vi "Logging Message Loop.vi"(8 "error in (no error)":errorcluster, 10 "Data Queue":refnum<queue>, 11 "Message Queues":T1) -> (0 "error out":errorcluster)   [LabVIEW 2016, in "Logging.lvlib"]
doc: "The message loop subVI to handle messages pertaining to logging data."
uses:
  Logging.lvlib
  support/Message Queue/All Message Queues.ctl
  support/Message Queue/Message Cluster.ctl
  Logging Configuration.ctl
  Logging State.ctl
  support/Message Queue/Enqueue Message (Single).vi
  <vilib>/Utility/error.llb/Error Cluster From Error Code.vi
  <vilib>/ErrorRing/Error Ring.xnode
  support/Message Queue/Message Queue.lvlib
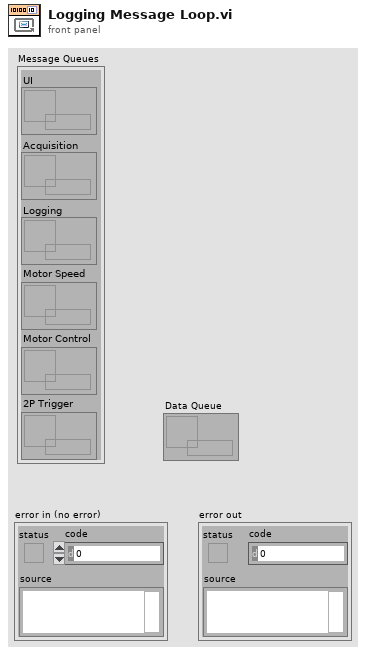
[diagram p1: front panel]
types:
  T1 = typedef "Message Queue.lvlib/All Message Queues.ctl" = cluster{"UI":refnum<queue>, "Acquisition":refnum<queue>, "Logging":refnum<queue>, "Motor Speed":refnum<queue>, "Motor Control":refnum<queue>, "2P Trigger":refnum<queue>}
  T2 = typedef "Logging.lvlib/Logging State.ctl" = cluster{"State":enum16{"Logging", "Not Logging", "Idle"}, "Samples to Save":u32, "Force Trigger":bool}
  T3 = typedef "Logging.lvlib/Logging Configuration.ctl" = cluster{"Log File Base Path":path, "TDMS File Reference":refnum<k34>, "Samples to Save":u32, "Trigger - Time":u32, "Trigger - Threshold":dbl, "Trigger - Channel":u32, "Enable Time Trigger":bool, "Enable Threshold Trigger":bool, "Always Log":bool}
  T4 = enum16{"open", "open or create", "create or replace", "create", "open (read-only)"}
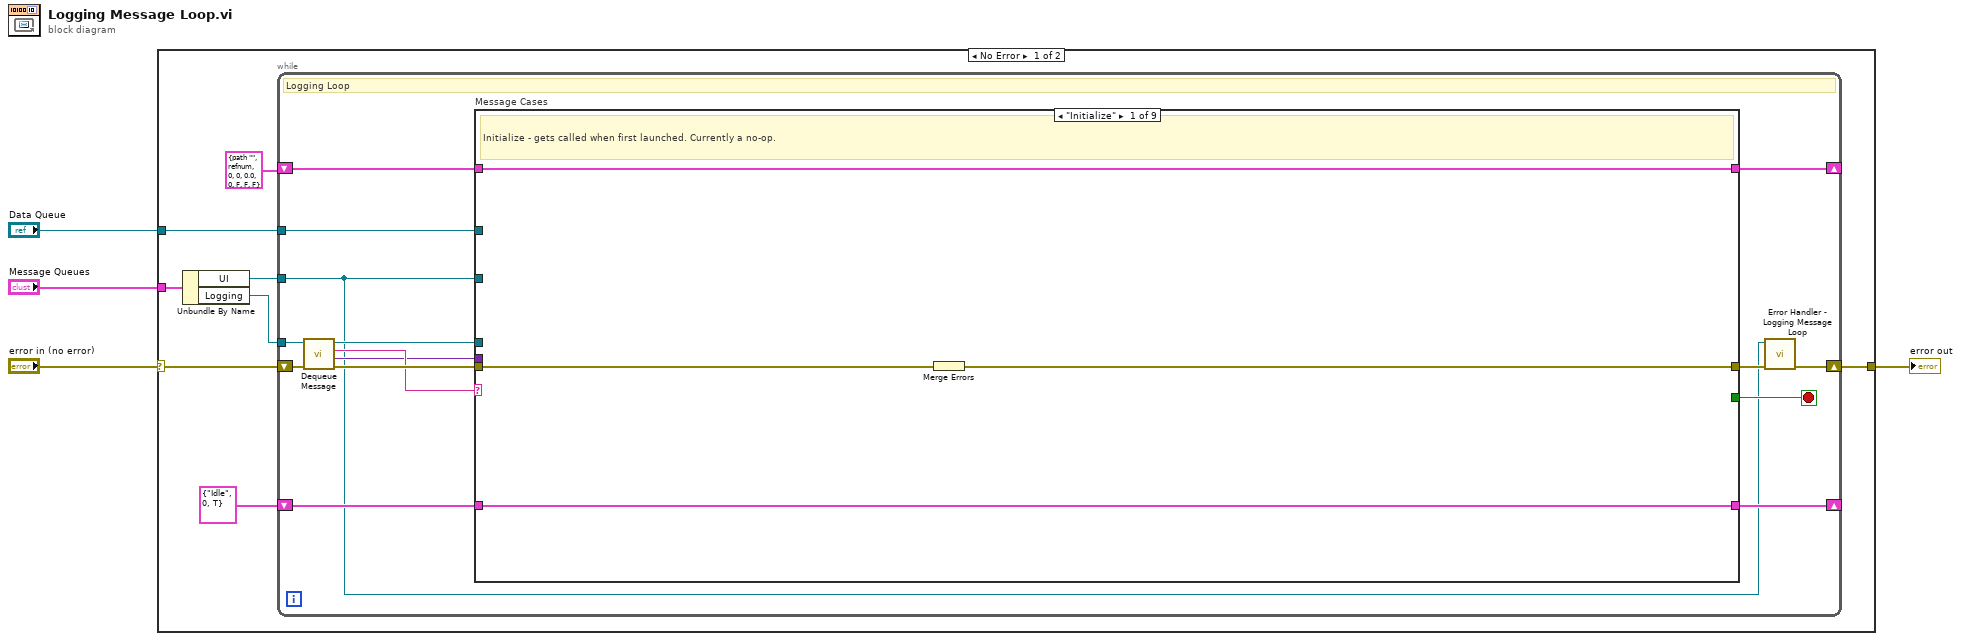
[diagram p0: block diagram]
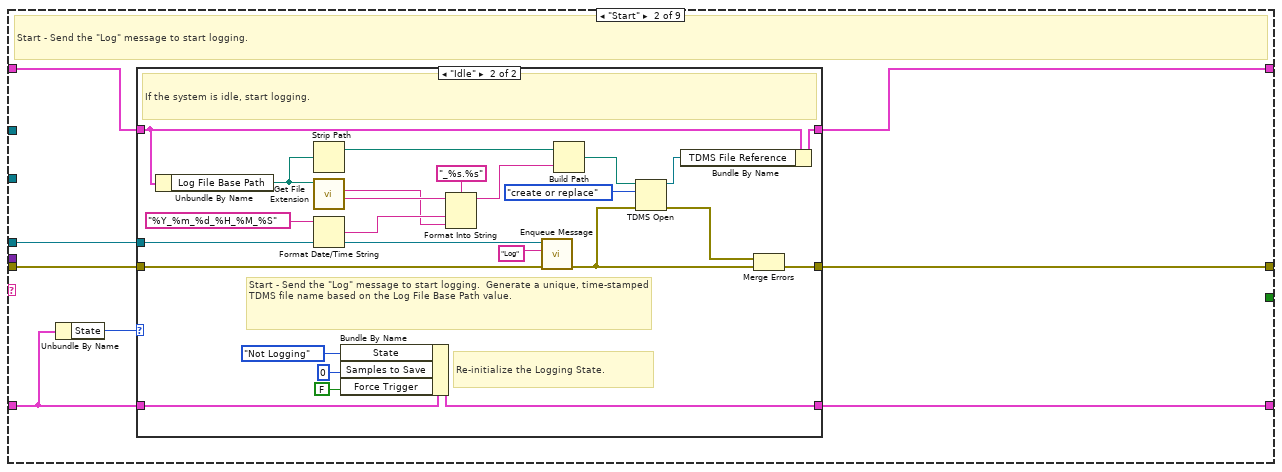
[diagram p2: hidden frame]
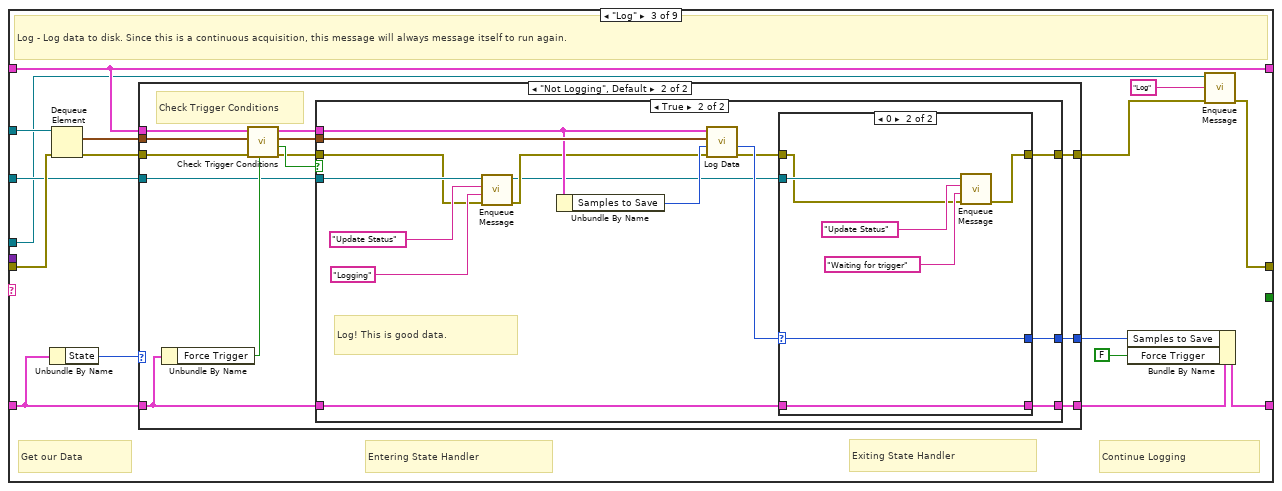
[diagram p4: hidden frame]
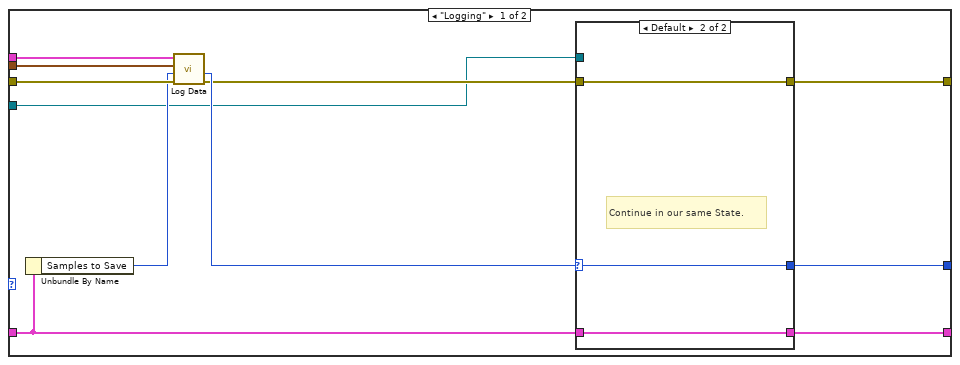
[diagram p5: hidden frame]
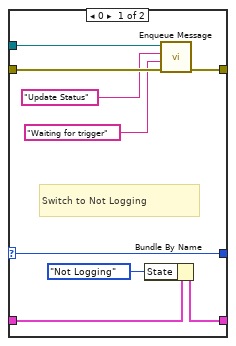
[diagram p6: hidden frame]
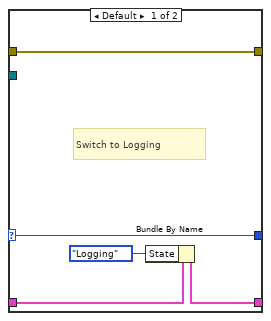
[diagram p8: hidden frame]
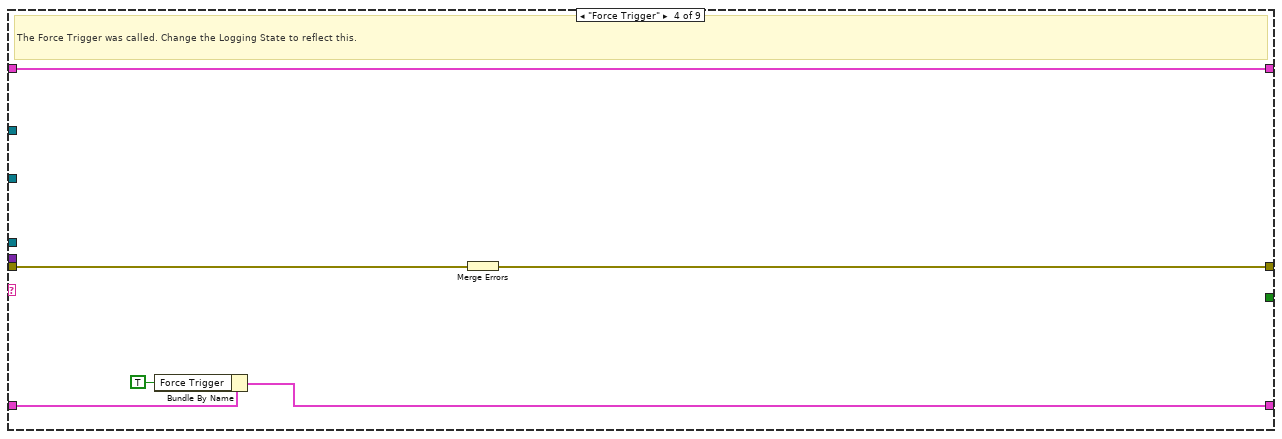
[diagram p9: hidden frame]
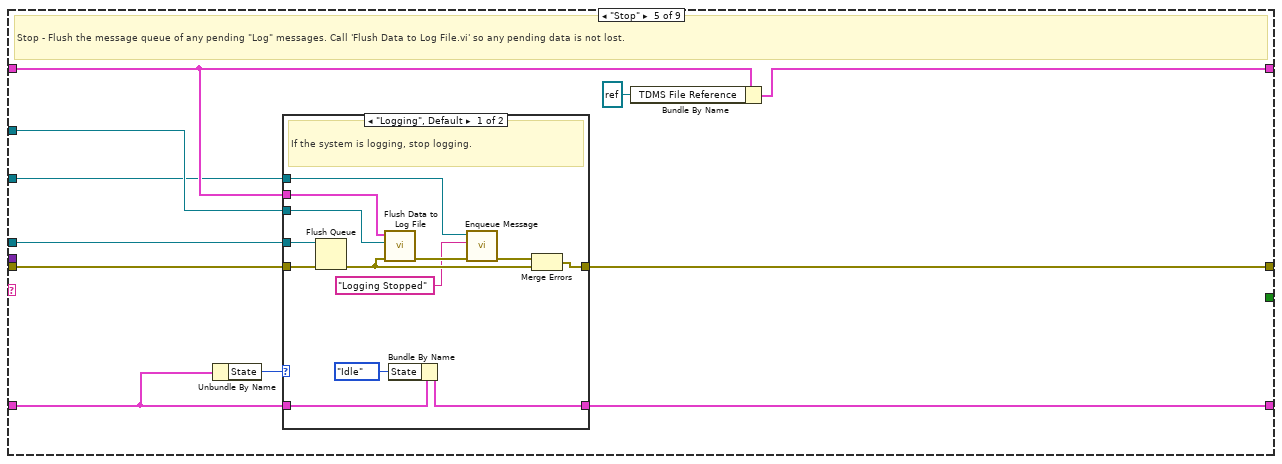
[diagram p10: hidden frame]
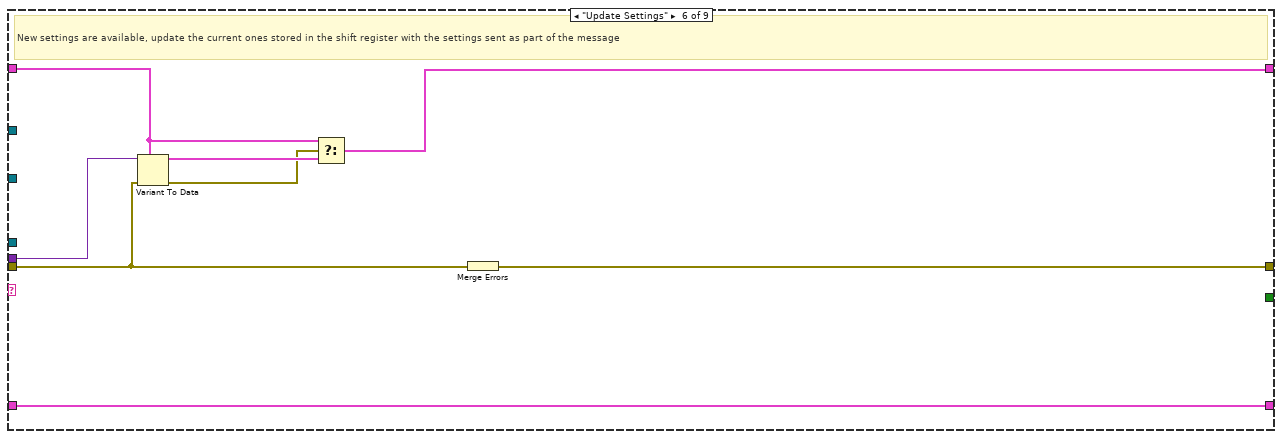
[diagram p12: hidden frame]
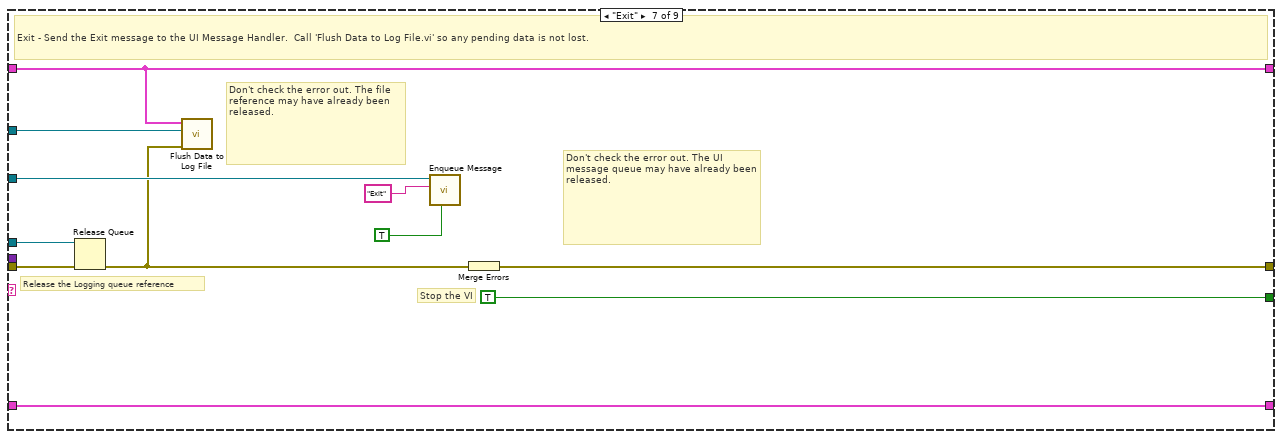
[diagram p13: hidden frame]
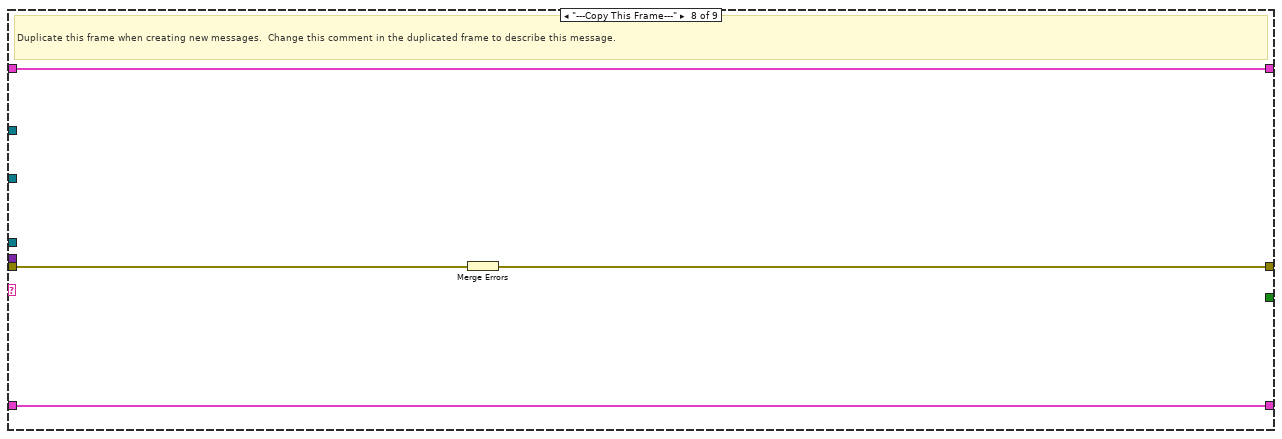
[diagram p14: hidden frame]
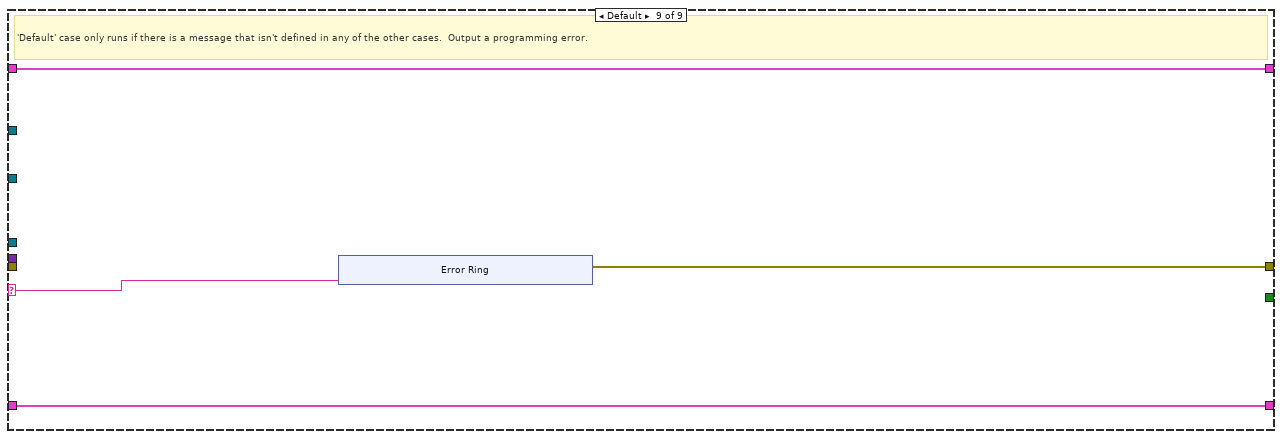
[diagram p15: hidden frame]
diagram:
  n1 = case shown="No Error" "error in (no error)" {
    selector: "error in (no error)" -> [w8 w214]
    tunnel: "Message Queues" -> [w12 _]
    tunnel: [w10 w214] -> w3
    tunnel: "Data Queue" -> [w7 _]
    frame No Error {
      n2 = Unbundle By Name(w12) -> ("UI"=w6:refnum<queue>, "Logging"=w11:refnum<queue>)
      n3 = while {
        tunnel: w11 -> [w19]
        shift-right: [w26] -> _
        shift-left: T3 {"Log File Base Path"=path "", "TDMS File Reference"=refnum, "Samples to Save"=0, "Trigger - Time"=0, "Trigger - Threshold"=0.0, "Trigger - Channel"=0, "Enable Time Trigger"=FALSE, "Enable Threshold Trigger"=FALSE, "Always Log"=FALSE} ("Logging Configuration") -> [w27]
        shift-right: [w14] -> w10
        shift-left: w8 -> [w24]
        tunnel: w6 -> [w13]
        tunnel: w7 -> [w18]
        shift-right: [w16] -> _
        shift-left: T2 {"State"=enum."Idle", "Samples to Save"=0, "Force Trigger"=TRUE} -> [w17]
        stop <- w25 stop-if-true
        # "Logging Loop"
        n4 = call "Dequeue Message.vi"("error in (no error)"=w24, "Message Queue"=w19) -> ("error out"=w23:errorcluster, "Message Data"=w21:variant, "Message"=w22:string, "dup Message Queue"=w20:refnum<queue>)  [unwired: 6 in]
        n5 = case "Message Cases" shown="\"Initialize\"" w22 {
          selector: w22 -> [_ _ _ _ _ _ _ _ w203]
          tunnel: w20 -> [_ w38 w70 _ w162 _ w192 _ _]
          tunnel: w23 -> [w29 w37 w80 w153 w163 w181 w195 w202 _]
          tunnel: [w31 w39 w82 w151 w164 w187 w197 w200 w204] -> w15
          tunnel: w27 -> [w30 w36 w75 w152 w159 w185 w191 w201 w206]
          tunnel: [w30 w35 w75 w152 w161 w182 w191 w201 w206] -> w26
          tunnel: [_ _ _ _ _ _ TRUE _ _] -> w25
          tunnel: w21 -> [_ _ _ _ _ w186 _ _ _]
          tunnel: w13 -> [_ _ w74 _ w157 _ w196 _ _]
          tunnel: w18 -> [_ _ w71 _ w158 _ w190 _ _]
          tunnel: w17 -> [w28 w33 w78 w150 w155 w180 w188 w199 w205]
          tunnel: [w28 w34 w73 w149 w154 w180 w188 w199 w205] -> w16
          frame "Initialize" {
            # "Initialize - gets called when first launched. Currently a no-op."
            n6 = Merge Errors(w29) -> (w31:errorcluster)
          }
          frame "Start" {
            # "Start - Send the \"Log\" message to start logging."
            n7 = Unbundle By Name(w33) -> ("State"=w32:enum16{"Logging", "Not Logging", "Idle"})
            n8 = case shown="\"Idle\"" w32 {
              tunnel: [w41 w66] -> w39
              tunnel: w38 -> [_ w65]
              tunnel: w37 -> [w41 w63]
              tunnel: w36 -> [w42 w54]
              tunnel: [w42 w51] -> w35
              tunnel: w33 -> [w40 w47]
              tunnel: [w40 w46] -> w34
              frame "Logging", Default {
                # "The system is already running. Ignore the \"Start\" message."
              }
              frame "Idle" {
                # "Re-initialize the Logging State."
                # "Start - Send the \"Log\" message to start logging.  Generate a unique, time-stamped TDMS file name based on the Log File Base Path value."
                # "If the system is idle, start logging."
                n9 = Unbundle By Name(w54) -> ("Log File Base Path"=w61:path)
                n10 = Strip Path(path=w61) -> (stripped path=w60:path)  [unwired: 1 out]
                n11 = call <vilib>:"Get File Extension.vi"("file"=w61) -> ("filename without extension"=w59:string, "lowercase file extension"=w56:string)  [unwired: 6 in, 3 out]
                n12 = Format Date/Time String(time format string (%c)="%Y_%m_%d_%H_%M_%S") -> (date/time string=w57:string)  [unwired: 2 in]
                n13 = Bundle By Name(cluster=w47, "State"=enum16{"Logging", "Not Logging"}."Not Logging", "Samples to Save"=u32 0 ("Reads to Save"), "Force Trigger"=FALSE) -> (w46:T2)
                n14 = Format Into String(format string="_%s.%s", initial string=w59, w57, w56) -> (resulting string=w55:string)  [unwired: 1 in, 1 out]
                n15 = call-poly "Enqueue Message.vi"("error in (no error)"=w63, "Message"="Log", "Message Queue"=w65) -> ("error out"=w49:errorcluster)  [unwired: 7 in, 1 out]
                n16 = Build Path(base path=w60, name or relative path=w55) -> (appended path=w52:path)
                n17 = TDMS Open(8:w49, 10:T4."create or replace" ("operation (0:open)"), 11:w52) -> (0:w48:errorcluster, 3:w53:refnum<k34>)  [unwired: 4 in]
                n18 = Bundle By Name(cluster=w54, "TDMS File Reference"=w53) -> (w51:T3)
                n19 = Merge Errors(w48, w49) -> (w66:errorcluster)
              }
            }
          }
          frame "Log" {
            # "Exiting State Handler"
            # "Continue Logging"
            # "Entering State Handler"
            # "Get our Data"
            # "Log - Log data to disk. Since this is a continuous acquisition, this message will always message itself to run again."
            n20 = Unbundle By Name(w78) -> ("State"=w79:enum16{"Logging", "Not Logging", "Idle"})
            n21 = Dequeue Element(queue=w71, error in (no error)=w80) -> (element=w77:waveform(dbl)[], error out=w76:errorcluster)  [unwired: 1 in, 2 out]
            n22 = case shown="\"Not Logging\", Default" w79 {
              tunnel: [w87 w110] -> w69
              tunnel: w78 -> [w88 w108]
              tunnel: w77 -> [w92 w117]
              tunnel: w76 -> [w91 w116]
              tunnel: w75 -> [w93 w118]
              tunnel: w74 -> [w83 w107]
              tunnel: [w84 w109] -> w67
              tunnel: [w86 w106] -> w68
              frame "Logging" {
                n23 = Unbundle By Name(w88) -> ("Samples to Save"=w90:u32)
                n24 = call "Log Data.vi"("error in (no error)"=w91, "Samples to Save In"=w90, "Data"=w92, "Logging Configuration"=w93) -> ("error out"=w85:errorcluster, "Samples to Save Out"=w89:u32)  [unwired: 6 in]
                n25 = case shown="Default" w89 {
                  selector: w89 -> [w99 w105]
                  tunnel: w85 -> [w97 w104]
                  tunnel: [w98 w104] -> w84
                  tunnel: w88 -> [w101 w103]
                  tunnel: [w100 w103] -> w87
                  tunnel: [w99 w105] -> w86
                  tunnel: w83 -> [w94 _]
                  frame 0 {
                    # "Switch to Not Logging"
                    n26 = Bundle By Name(cluster=w101, "State"=enum16{"Logging", "Not Logging"}."Not Logging") -> (w100:T2)
                    n27 = call-poly "Enqueue Message.vi"("error in (no error)"=w97, "Message Data"="Waiting for trigger" ("Waiting for trigger"), "Message"="Update Status", "Message Queue"=w94) -> ("error out"=w98:errorcluster)  [unwired: 6 in, 1 out]
                  }
                  frame Default {
                    # "Continue in our same State."
                  }
                }
              }
              frame "Not Logging", Default {
                # "Check Trigger Conditions"
                n28 = Unbundle By Name(w108) -> ("Force Trigger"=w115:bool)
                n29 = call "Check Trigger Conditions.vi"("Force Trigger?"=w115, "error in (no error)"=w116, "Waveform Data In"=w117, "Logging Configuration In"=w118) -> ("error out"=w113:errorcluster, "Trigger Conditions Met?"=w114:bool, "Waveform Data Out (copy)"=w112:waveform(dbl)[], "Logging Configuration Out"=w111:T3)  [unwired: 4 in]
                n30 = case shown="True" w114 {
                  tunnel: w113 -> [w119 w129]
                  tunnel: w112 -> [_ w135]
                  tunnel: w111 -> [_ w134]
                  tunnel: w108 -> [w120 w125]
                  tunnel: [w120 w124] -> w110
                  tunnel: [w119 w122] -> w109
                  tunnel: w107 -> [_ w133]
                  tunnel: [_ w126] -> w106
                  frame False {
                  }
                  frame True {
                    # "Log! This is good data."
                    n31 = call-poly "Enqueue Message.vi"("error in (no error)"=w129, "Message Data"="Logging" ("Logging"), "Message"="Update Status", "Message Queue"=w133) -> ("error out"=w128:errorcluster, "dup Message Queue"=w121:refnum<queue>)  [unwired: 6 in]
                    n32 = Unbundle By Name(w134) -> ("Samples to Save"=w130:u32)
                    n33 = call "Log Data.vi"("error in (no error)"=w128, "Samples to Save In"=w130, "Data"=w135, "Logging Configuration"=w134) -> ("error out"=w123:errorcluster, "Samples to Save Out"=w127:u32)  [unwired: 6 in]
                    n34 = case shown="0" w127 {
                      selector: w127 -> [w140 w147]
                      tunnel: [w140 w147] -> w126
                      tunnel: [w137 w146] -> w124
                      tunnel: w125 -> [w138 w146]
                      tunnel: w123 -> [w136 w142]
                      tunnel: [w136 w141] -> w122
                      tunnel: w121 -> [_ w145]
                      frame Default {
                        # "Switch to Logging"
                        n35 = Bundle By Name(cluster=w138, "State"=enum16{"Logging", "Not Logging"}."Logging") -> (w137:T2)
                      }
                      frame 0 {
                        n36 = call-poly "Enqueue Message.vi"("error in (no error)"=w142, "Message Data"="Waiting for trigger" ("Waiting for trigger"), "Message"="Update Status", "Message Queue"=w145) -> ("error out"=w141:errorcluster)  [unwired: 6 in, 1 out]
                      }
                    }
                  }
                }
              }
            }
            n37 = Bundle By Name(cluster=w69, "Samples to Save"=w68, "Force Trigger"=FALSE) -> (w73:T2)
            n38 = call-poly "Enqueue Message.vi"("error in (no error)"=w67, "Message"="Log", "Message Queue"=w70) -> ("error out"=w82:errorcluster)  [unwired: 7 in, 1 out]
          }
          frame "Force Trigger" {
            # "The Force Trigger was called. Change the Logging State to reflect this."
            n39 = Bundle By Name(cluster=w150, "Force Trigger"=TRUE) -> (w149:T2)
            n40 = Merge Errors(w153) -> (w151:errorcluster)
          }
          frame "Stop" {
            # "Stop - Flush the message queue of any pending \"Log\" messages. Call 'Flush Data to Log File.vi' so any pending data is not lost."
            n41 = Unbundle By Name(w155) -> ("State"=w156:enum16{"Logging", "Not Logging", "Idle"})
            n42 = case shown="\"Logging\", Default" w156 {
              tunnel: [w177 w179] -> w164
              tunnel: w163 -> [w176 w179]
              tunnel: w162 -> [w175 _]
              tunnel: w159 -> [w174 _]
              tunnel: w158 -> [w173 _]
              tunnel: w157 -> [w169 _]
              tunnel: w155 -> [w167 w178]
              tunnel: [w166 w178] -> w154
              frame "Logging", Default {
                # "If the system is logging, stop logging."
                n43 = Flush Queue(queue=w175, error in (no error)=w176) -> (error out=w172:errorcluster)  [unwired: 2 out]
                n44 = call "Flush Data to Log File.vi"("error in (no error)"=w172, "Data Queue"=w173, "Logging Configuration"=w174) -> ("error out"=w171:errorcluster)  [unwired: 8 in]
                n45 = Bundle By Name(cluster=w167, "State"=enum16{"Logging", "Not Logging", "Idle"}."Idle") -> (w166:T2)
                n46 = call-poly "Enqueue Message.vi"("error in (no error)"=w171, "Message"="Logging Stopped", "Message Queue"=w169) -> ("error out"=w170:errorcluster)  [unwired: 7 in, 1 out]
                n47 = Merge Errors(w170, w172) -> (w177:errorcluster)
              }
              frame "Idle" {
                # "The system is already idle. Ignore the \"Stop\" message."
              }
            }
            n48 = Bundle By Name(cluster=w159, "TDMS File Reference"=refnum<k34> refnum ("tdms file out")) -> (w161:T3)
          }
          frame "Update Settings" {
            # "New settings are available, update the current ones stored in the shift register with the settings sent as part of the message"
            n49 = Variant To Data(error in=w181, type=w185, Variant=w186) -> (data=w184:T3, error out=w183:errorcluster)
            n50 = Select(t=w185, s=w183, f=w184) -> (s? t:f=w182:T3)
            n51 = Merge Errors(w181) -> (w187:errorcluster)
          }
          frame "Exit" {
            # "Don't check the error out. The file reference may have already been released."
            # "Release the Logging queue reference"
            # "Don't check the error out. The UI message queue may have already been released."
            # "Stop the VI"
            # "Exit - Send the Exit message to the UI Message Handler.  Call 'Flush Data to Log File.vi' so any pending data is not lost."
            n52 = Release Queue(queue=w192, error in (no error)=w195) -> (error out=w189:errorcluster)  [unwired: 1 in, 2 out]
            n53 = call "Flush Data to Log File.vi"("error in (no error)"=w189, "Data Queue"=w190, "Logging Configuration"=w191) -> ()  [unwired: 8 in, 1 out]
            n54 = call-poly "Enqueue Message.vi"("Priority Message? (F)"=TRUE, "Message"="Exit", "Message Queue"=w196) -> ()  [unwired: 7 in, 2 out]
            n55 = Merge Errors(w189) -> (w197:errorcluster)
          }
          frame "---Copy This Frame---" {
            # "Duplicate this frame when creating new messages.  Change this comment in the duplicated frame to describe this message."
            n56 = Merge Errors(w202) -> (w200:errorcluster)
          }
          frame Default {
            # "'Default' case only runs if there is a message that isn't defined in any of the other cases.  Output a programming error."
            n57 = xnode "Error Ring"("parameter 0"=w203) -> ("error out"=w204:errorcluster)
          }
        }
        n58 = call "Error Handler - Logging Message Loop.vi"("error in (no error)"=w15, "Message Queue"=w13) -> ("dup error in"=w14:errorcluster)  [unwired: 8 in, 1 out]
      }
    }
    frame Error {
    }
  }
  "error out" <- w3
